vi "GetTCPanel.vi"(6 "错误输入（无错误）":errorcluster, 9 "机器名(\"\": 打开本地引用)":string="10.215.142.232") -> (0 "错误输出":errorcluster, 3 "Panel":refnum<vi>)   [LabVIEW 2017]
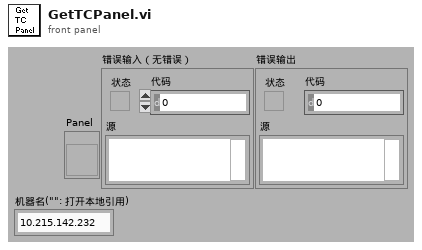
[diagram p1: front panel]
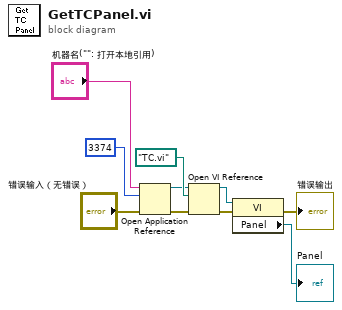
[diagram p0: block diagram]
diagram:
  n1 = Open Application Reference(8:"错误输入（无错误）", 10:u16 3374 ("端口号或服务名称(3363)"), 11:"机器名(\"\": 打开本地引用)") -> (0:w4:errorcluster, 3:w7:refnum<vi>)  [unwired: 1 out]
  n2 = Open VI Reference(application reference (local)=w7, vi path=path "TC.vi" ("VI路径"), error in (no error)=w4) -> (vi reference=w9:refnum<vi>, error out=w3:errorcluster)  [unwired: 3 out]
  n3 = property class="VI"(reference=w9, error in=w3) -> (error out=→"错误输出":errorcluster, "Panel"=→"Panel":refnum<vi>)  [unwired: 1 out]
